vi "SA Cond - Concatenate Signals.vi"(0 "Signal IN":waveform(dbl)[](array[waveform]), 5 "error in (no error)":errorcluster, 6 "Anotate Signal Name":bool=TRUE) -> (14 "Signal OUT":waveform(dbl)[](array[waveform]), 19 "error out":errorcluster)   [LabVIEW 2020, in "GSwFormDSP.lvclass"]
uses:
  GSwFormDSP.lvclass
  Attribute List.ctl
  Attribute Options.ctl
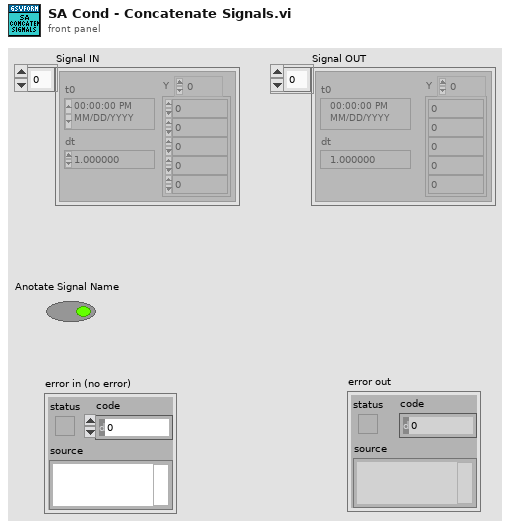
[diagram p1: front panel]
types:
  T1 = typedef "GSwFormDSP.lvclass/Attribute List.ctl" = string
  T2 = typedef "GSwFormDSP.lvclass/Attribute Options.ctl" = enum16{"Append to Attribute using \"( )\"", "Replace Attribute Value"}
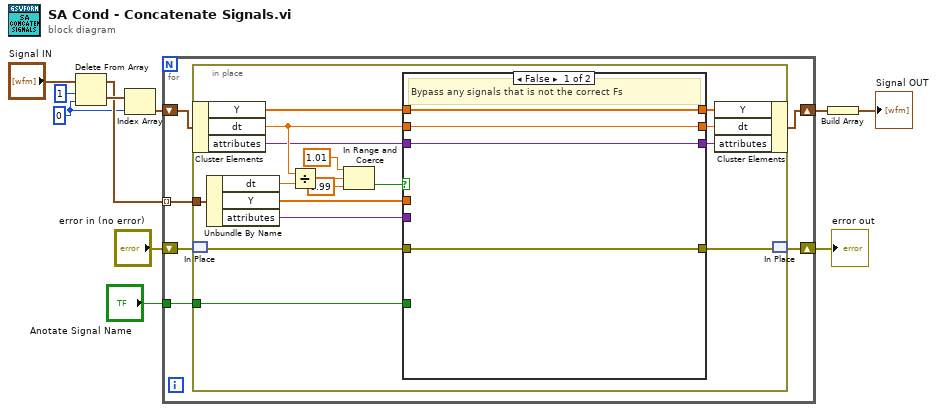
[diagram p0: block diagram]
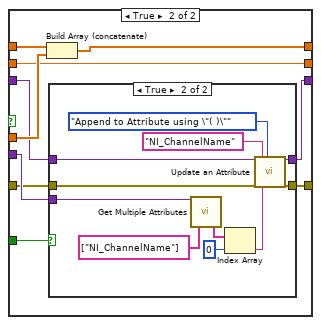
[diagram p2: hidden frame]
diagram:
  w5 = 0 ("index")
  n1 = Delete From Array(array="Signal IN", length=1, index=w5) -> (deleted portion=w8:waveform(dbl)[], array with subset deleted=w6:waveform(dbl)[])
  n2 = Index Array(array=w8, index=w5) -> (element=w7:waveform(dbl))
  n3 = for {
    shift-right: [w15] -> w4
    shift-left: w7 -> [w17]
    tunnel: w6 -> [w16] mode=indexing
    tunnel: "Anotate Signal Name" -> [w14]
    shift-right: [w12] -> w1
    shift-left: "error in (no error)" -> [w13]
    n4 = in-place {
      in-place-border: w16 -> [w33]
      in-place-border: w14 -> [w24]
      n5 = in-place-cluster #1(w17) -> ("Y"=w34:dbl[], "dt"=w28:dbl, "attributes"=w27:variant)
      n6 = in-place-match #2(w13) -> (w23:errorcluster)
      n7 = Unbundle By Name(w33) -> ("dt"=w32:dbl, "Y"=w31:dbl[], "attributes"=w25:variant)
      n8 = Divide(x=w28, y=w32) -> (x/y=w21:dbl)
      n9 = In Range and Coerce(upper limit=1.01, x=w21, lower limit=0.99) -> (In Range?=w20:bool)  [unwired: 1 out]
      n10 = case shown="False" w20 {
        tunnel: w34 -> [w38 w48]
        tunnel: w31 -> [_ w47]
        tunnel: [w38 w46] -> w30
        tunnel: [w37 w45] -> w29
        tunnel: w28 -> [w37 w45]
        tunnel: w27 -> [w36 w44]
        tunnel: [w36 w42] -> w26
        tunnel: w25 -> [_ w43]
        tunnel: w24 -> [_ w41]
        tunnel: w23 -> [w35 w40]
        tunnel: [w35 w39] -> w22
        frame False {
          # "Bypass any signals that is not the correct Fs"
        }
        frame True {
          n11 = Build Array (concatenate)(w48, w47) -> (w46:dbl[])
          n12 = case shown="True" w41 {
            tunnel: w44 -> [w50 w61]
            tunnel: [w50 w60] -> w42
            tunnel: w43 -> [_ w59]
            tunnel: w40 -> [w49 w52]
            tunnel: [w49 w51] -> w39
            frame False {
            }
            frame True {
              n13 = call "Get Multiple Attributes.vi"("Attributes IN"=w59, "Attribute List"=T1[] ["NI_ChannelName"]) -> ("Values"=w57:string[])  [unwired: 16 in, 1 out]
              n14 = Index Array(array=w57, index=0) -> (element=w55:string)
              n15 = call "Update an Attribute.vi"("attributes in"=w61, "error in (no error)"=w52, "Attribute List"=T1 "NI_ChannelName", "Attribute Value"=w55, "Attribute Option"=Attribute_Options."Append to Attribute using \"( )\"") -> ("attributes out"=w60:variant, "error out"=w51:errorcluster)  [unwired: 13 in]
            }
          }
        }
      }
      n16 = in-place-cluster #1("Y"=w30, "dt"=w29, "attributes"=w26) -> (w15:waveform(dbl))
      n17 = in-place-match #2(w22) -> (w12:errorcluster)
    }
  }
  "error out" <- w1
  n18 = Build Array(w4) -> (→"Signal OUT":waveform(dbl)[])
